vi "createDough.vi"(8 "error in (no error)":errorcluster, 11 "ChicagoPizzaIngredientFactory in":refnum<class "ChicagoPizzaIngredientFactory.lvclass">) -> (0 "error out":errorcluster, 2 "Ingredients":string, 3 "ChicagoPizzaIngredientFactory out":refnum<class "ChicagoPizzaIngredientFactory.lvclass">)   [LabVIEW 2013, in "ChicagoPizzaIngredientFactory.lvclass"]
uses:
  ChicagoPizzaIngredientFactory.lvclass
  ChicagoPizzaIngredientFactory.lvclass/ChicagoPizzaIngredientFactory.ctl
  Dough.lvclass/Dough.lvclass
panel:
  # "產出麵皮"
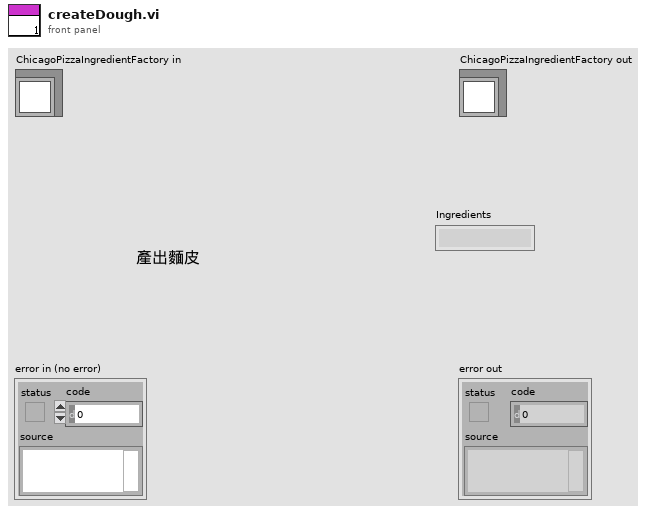
[diagram p1: front panel]
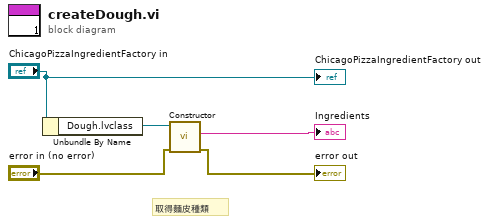
[diagram p0: block diagram]
diagram:
  # "取得麵皮種類"
  n1 = Unbundle By Name("ChicagoPizzaIngredientFactory in") -> ("Dough.lvclass"=w4:refnum<class "Dough.lvclass">)
  n2 = call-dynamic "Constructor.vi"("error in (no error)"="error in (no error)", "Dough in"=w4) -> ("error out"=→"error out":errorcluster, "Ingredients"=→"Ingredients":string)  [unwired: 7 in, 1 out]
  "ChicagoPizzaIngredientFactory out" <- "ChicagoPizzaIngredientFactory in"
